vi "LS336_Setpoint_Status_DP_ver1.0.vi"(4 "error in":errorcluster, 5 "Mode: (default: 2)":i16(ring)=2 items=["Do nothing to mark the end of the transfer", "Send NL (linefeed) with EOI after the data bytes.", "Send EOI with the last data byte in the string(default)"], 6 "Output's control loop (1)":i32=1, 7 "GPIB ADR (18)":i16=18) -> (0 "error out":errorcluster, 1 "SetPoint":string, 2 "Setpoint":dbl, 3 "dump GPIB ADR":i16)   [LabVIEW 2012]
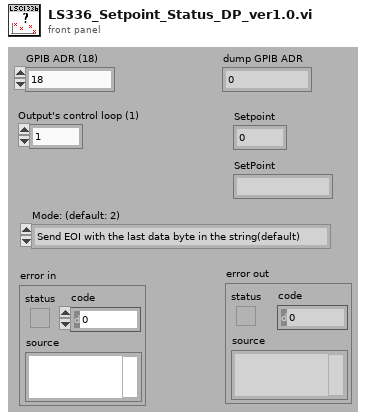
[diagram p1: front panel]
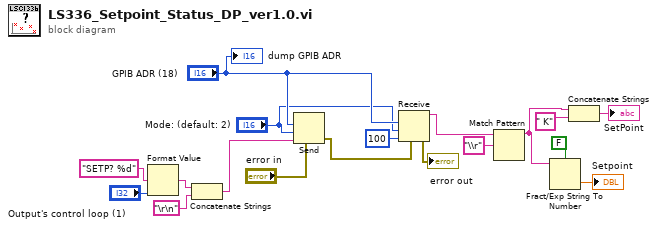
[diagram p0: block diagram]
diagram:
  n1 = Format Value(format string="SETP? %d", value (0)="Output's control loop (1)") -> (output string=w16:string)  [unwired: 1 out]
  n2 = Concatenate Strings(w16, "\r\n") -> (w14:string)
  n3 = Send(2:"GPIB ADR (18)", 3:"Mode: (default: 2)", 4:"error in", 5:w14) -> (8:w12:errorcluster)  [unwired: 1 in, 2 out]
  n4 = Receive(4:w12, 6:100 ("count"), 7:"Mode: (default: 2)", 8:"GPIB ADR (18)") -> (0:→"error out":errorcluster, 3:w8:string)  [unwired: 3 out]
  n5 = Match Pattern(string=w8, regular expression="\\r") -> (before substring=w2:string)  [unwired: 4 out]
  n6 = Fract/Exp String To Number(use system decimal point (T)=FALSE, string=w2) -> (number=→"Setpoint":dbl)  [unwired: 3 out]
  n7 = Concatenate Strings(w2, " K" ("string")) -> (→"SetPoint":string)
  "dump GPIB ADR" <- "GPIB ADR (18)"
